vi "IT7800 Open.vi"(8 "error in":errorcluster, 11 "IP Address":string="192.168.0.252") -> (0 "error out":errorcluster, 3 "VISA out":refnum<visa-resource-name>)   [LabVIEW 2025]
uses:
  <instrlib>/IT7800/IT7800.lvlib
panel:
  # "Note: Measure filter to ON, default measure rate of 500ms, Input1 as SafetyOFF"
  # "IP7800 Driver V0.11\nOpen"
  # "19.05.2025"
  # "Andrej Valand"
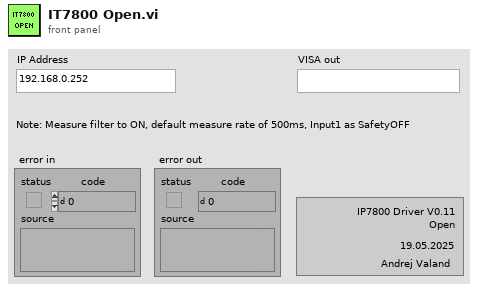
[diagram p1: front panel]
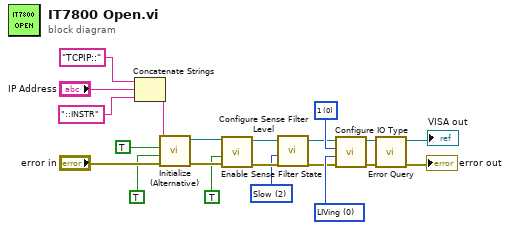
[diagram p0: block diagram]
diagram:
  w6 = u8 0 items=["LIVing", "LATCh", "PSCLear", "PSSTate", "SYIN", "SYOut", "OFFState", "TIN1", "TIN2", "TOUT1", "TOUT2", "IORD", "IOWR"] ("Type")
  w7 = u8 0 items=["1", "2", "3", "4", "5", "6", "7"] ("IO")
  w9 = u8 2 items=["Lowest", "Lower", "Slow", "Medium", "Fast"] ("Type")
  n1 = Concatenate Strings("TCPIP::" ("string"), "IP Address", "::INSTR" ("string")) -> (w16:string)
  n2 = call "Initialize (Alternative).vi"("error in"="error in", "Reset"=TRUE, "ID Query"=TRUE, "VISA resource name"=w16) -> ("error out"=w12:errorcluster, "VISA resource name out"=w15:refnum<visa-resource-name>)  [unwired: 6 in]
  n3 = call <instrlib>:"Enable Sense Filter State.vi"("error in"=w12, "State"=TRUE, "VISA resource name"=w15) -> ("error out"=w11:errorcluster, "VISA resource name out"=w14:refnum<visa-resource-name>)  [unwired: 7 in]
  n4 = call <instrlib>:"Configure Sense Filter Level.vi"("error in"=w11, "Type"=w9, "VISA resource name"=w14) -> ("error out"=w3:errorcluster, "VISA resource name out"=w2:refnum<visa-resource-name>)  [unwired: 7 in]
  n5 = call <instrlib>:"Configure IO Type.vi"("error in"=w3, "Type"=w6, "IO"=w7, "VISA resource name"=w2) -> ("error out"=w4:errorcluster, "VISA resource name out"=w5:refnum<visa-resource-name>)  [unwired: 6 in]
  n6 = call <instrlib>:"Error Query.vi"("error in"=w4, "VISA resource name"=w5) -> ("error out"=→"error out":errorcluster, "VISA resource name out"=→"VISA out":refnum<visa-resource-name>)  [unwired: 6 in, 2 out]
